vi "Prep File.vi"(4 "Num Samps":i32, 5 "Num Segs":i32, 6 "File Name":string) -> (0 "File Handle":u32, 2 "refnum out":refnum<file>)   [LabVIEW 2022 SP3]
uses:
  ScanningControl/Motion Controllers/-MotionRoutines/MotionGlobals.vi
  <instrlib>/niHWS/nihws.llb/niHWS Open File Permissions ID.ctl
  <instrlib>/niHWS/nihws.llb/niHWS Write Analog WDT.vi
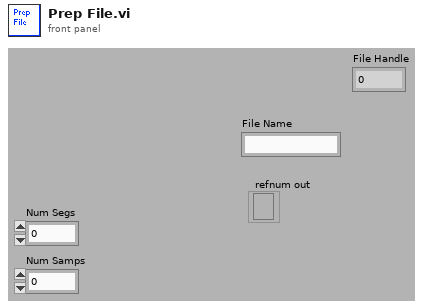
[diagram p1: front panel]
types:
  T1 = typedef "niHWS Open File Permissions ID.ctl" = enum32{"Read Only", "Read/Write Existing", "Read/Write/Create New", "Read/Write/Create New Always"}
  T2 = enum16{"open", "replace", "create", "open or create", "replace or create", "replace or create with confirmation"}
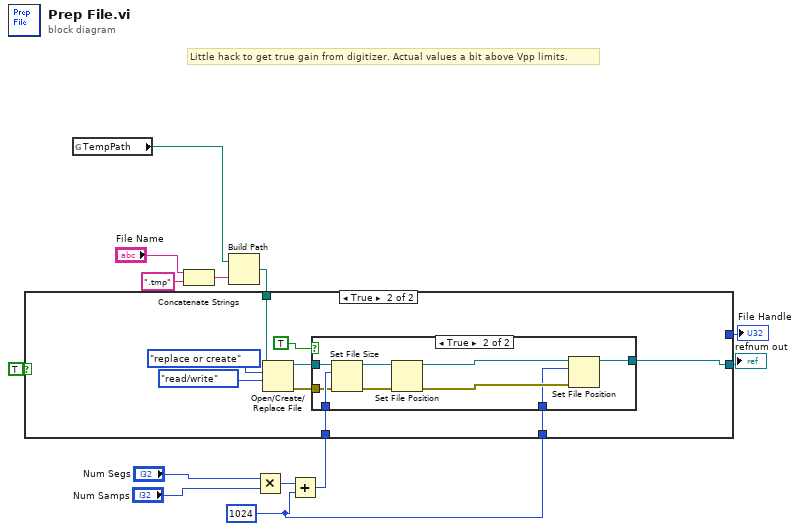
[diagram p0: block diagram]
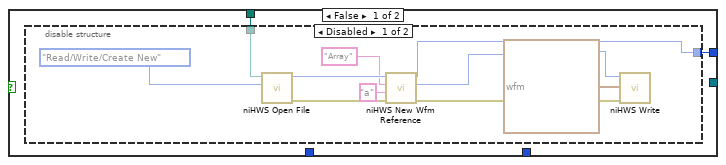
[diagram p2: hidden frame]
diagram:
  w2 = 1024
  # "Little hack to get true gain from digitizer. Actual values a bit above Vpp limits."
  n1 = global read "MotionGlobals.vi" "TempPath"() -> (w1:path)
  n2 = Concatenate Strings("File Name", ".tmp") -> (w8:string)
  n3 = Build Path(base path=w1, name or relative path=w8) -> (appended path=w6:path)
  n4 = Multiply(x="Num Segs", y="Num Samps") -> (x*y=w12:i32)
  n5 = Add(x=w12, y=w2) -> (x+y=w13:i32)
  n6 = case shown="True" TRUE {
    tunnel: w13 -> [_ w34]
    tunnel: [_ w27] -> w9
    tunnel: w6 -> [w15 w29]
    tunnel: [w14 _] -> w4
    tunnel: w2 -> [_ w28]
    frame False {
      n7 = disable-structure shown="Disabled" {
        disable-tunnel: w15 -> [w24 _]
        disable-tunnel: [w18 _] -> w14
        frame Disabled {
          n8 = call <instrlib>:"niHWS Open File.vi"("permissions (0:read only)"=niHWS_Open_File_Permissions_ID."Read/Write/Create New", "file path"=w24) -> ("error out"=w22:errorcluster, "file handle"=w23:u32)  [unwired: 1 in, 7 out]
          n9 = call <instrlib>:"niHWS New Wfm Reference.vi"("error in (no error)"=w22, "waveform name (empty)"="a", "group name (empty)"="Array", "file handle in"=w23) -> ("error out"=w21:errorcluster, "waveform reference"=w19:u32, "file handle out"=w18:u32)  [unwired: 1 in, 4 out]
          n10 = call-poly <instrlib>:"niHWS Write.vi"("error in (no error)"=w21, "analog waveform"=waveform(dbl) {"t0"=timestamp(0 s since 1904-01-01), "dt"=0.0, "Y"=[]}, "waveform reference in"=w19) -> ()  [unwired: 9 out]
        }
        frame Enabled {
        }
      }
    }
    frame True {
      n11 = Open/Create/Replace File(file path (use dialog)=w29, operation (0:open)=T2."replace or create", access (0:read/write)=enum16{"read/write", "read-only", "write-only"}."read/write") -> (refnum out=w32:refnum<file>, error out=w33:errorcluster)  [unwired: 1 in, 3 out]
      n12 = case shown="True" TRUE {
        tunnel: w34 -> [_ w44]
        tunnel: w33 -> [_ w43]
        tunnel: w32 -> [w35 w42]
        tunnel: w28 -> [_ w39]
        tunnel: [w35 w38] -> w27
        frame False {
        }
        frame True {
          n13 = Set File Size(4:w43, 6:w44, 7:w42) -> (0:w37:errorcluster, 3:w36:refnum<file>)
          n14 = Set File Position(refnum=w36, error in=w37) -> (refnum out=w41:refnum<file>, error out=w40:errorcluster)  [unwired: 1 in, 1 out]
          n15 = Set File Position(offset (in bytes) (0)=w39, refnum=w41, error in=w40) -> (refnum out=w38:refnum<file>)  [unwired: 1 in, 1 out]
        }
      }
    }
  }
  "refnum out" <- w9
  "File Handle" <- w4
